vi "setSweep.vi"(4 "sweep type (0 : linear)":T1, 6 "Number of Points":i32, 8 "error in (no error)":errorcluster, 9 "Stop (Hz)":dbl, 10 "Start (Hz)":dbl, 11 "Instrument.VSource in":refnum<class "Instrument.VNA.lvclass">) -> (0 "error out":errorcluster, 3 "Instrument.VSource out":refnum<class "Instrument.VNA.lvclass">)   [LabVIEW 2019, in "Instrument.VNA.lvclass"]
uses:
  Instrument.VNA.lvclass
  C:/Users/patrick/Documents/GitHub/Instrument-Framework/lvsrc/Instrument/Instrument.lvclass
  Typedefs/Sweep Type--enum.ctl
  Typedefs/setSweep--cluster.ctl
  6995be2c-71c1-44d3-a7f6-e9bca5642cdb.vi
  6995be2c-71c1-44d3-a7f6-e9bca5642cdb.vi/930d3bdd-9a03-4928-9faf-c08dfdfeff50.vi
  6995be2c-71c1-44d3-a7f6-e9bca5642cdb.vi/930d3bdd-9a03-4928-9faf-c08dfdfeff50.vi/fbd87a07-efa7-4932-8754-3ee77433eac6.vi
  6995be2c-71c1-44d3-a7f6-e9bca5642cdb.vi/930d3bdd-9a03-4928-9faf-c08dfdfeff50.vi/91e3e15a-bdb6-4351-9fd5-2baddd306962.vi
  Instrument/Private/Get RC Connection Status.vi
  Instrument/API/Send and Receive.vi
  <vilib>/Utility/Data Type/Get Type Information.vi
  <vilib>/JDP Science/JSONtext/JSON text to Variant.vi
  <vilib>/JDP Science/JSONtext/LVClass Serializer/JSONtext LVClass Serializer.lvclass
  Instrument/Instrument.lvclass
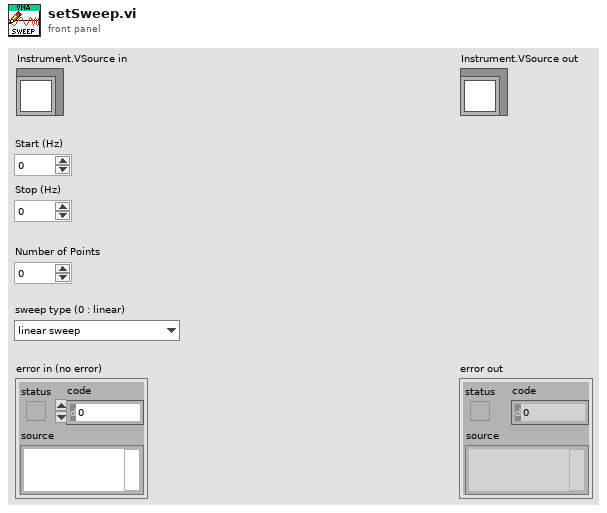
[diagram p1: front panel]
types:
  T1 = typedef "Instrument.VNA.lvclass/Sweep Type--enum.ctl" = enum16{"linear sweep", "logarithmic sweep", "frequency list", "CW time sweep", "power sweep"}
  T2 = typedef "Instrument.VNA.lvclass/setSweep--cluster.ctl" = cluster{"start":dbl, "stop":dbl, "points":i32, "type":T1}
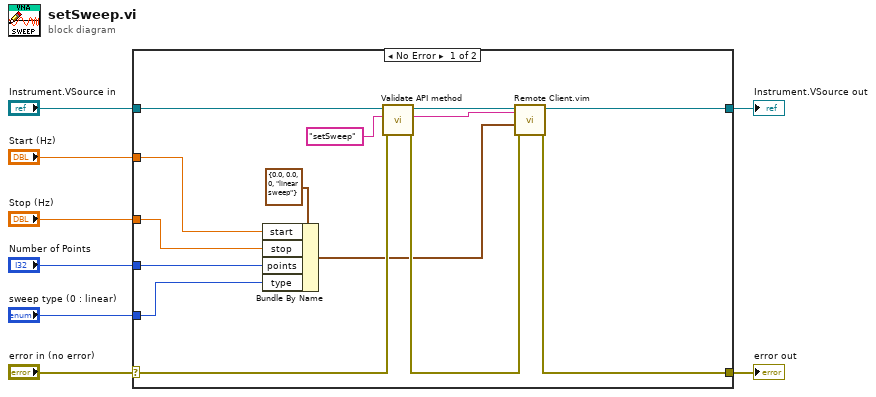
[diagram p0: block diagram]
diagram:
  n1 = case shown="No Error" "error in (no error)" {
    selector: "error in (no error)" -> [w17 w24]
    tunnel: [w15 w24] -> w7
    tunnel: [w18 w23] -> w5
    tunnel: "Instrument.VSource in" -> [w19 w23]
    tunnel: "Start (Hz)" -> [w10 _]
    tunnel: "Stop (Hz)" -> [w13 _]
    tunnel: "Number of Points" -> [w12 _]
    tunnel: "sweep type (0 : linear)" -> [w11 _]
    frame No Error {
      n2 = Bundle By Name(cluster=T2 {"start"=0.0, "stop"=0.0, "points"=0, "type"=enum."linear sweep"} ("setSweep"), "start"=w10, "stop"=w13, "points"=w12, "type"=w11) -> (w9:T2)
      n3 = call "Validate API method.vi"("error in (no error)"=w17, "Command in"="setSweep" ("error message (\"\")"), "Instrument in"=w19) -> ("error out"=w16:errorcluster, "command out"=w21:string, "Instrument out"=w20:refnum<class "Instrument.VNA.lvclass">)  [unwired: 6 in]
      n4 = call "Remote Client.vim"("Data Out type"=w21, "error in (no error)"=w16, "Data in"=w9, "Instrument in"=w20) -> ("error out"=w15:errorcluster, "Instrument out"=w18:refnum<class "Instrument.VNA.lvclass">)  [unwired: 4 in, 2 out]
    }
    frame Error {
    }
  }
  "error out" <- w7
  "Instrument.VSource out" <- w5
